vi "Acquire Data using 5772 (DRAM_sim).vi"() -> ()   [LabVIEW 2012]
uses:
  <vilib>/Platform/TimedLoop/XDataNode/XDataNode.xnode
  <vilib>/Platform/TimedLoop/XDataNode/nitl_modes.ctl
  <vilib>/Platform/TimedLoop/XDataNode/XDNodeRunTimeDep.lvlib
  <vilib>/Platform/TimedLoop/XDataNode/wakeup.ctl
  <vilib>/Platform/TimedLoop/XDataNode/timing_clust.ctl
  <vilib>/rvi/FXPMathLib/basic elements/FxpDiscreteDelay/XNode/nifxpmath_DiscreteDelay.xnode
  <userlib>/FPGA Library/Code Development/DRAM/RF-RIO/FIFO/FIFO/FPGA/FIFO.lvlib
  <userlib>/Fast OCT/Debug/Version 1/Channel Data/Data from Channel 0 and Channel 1.vi
  <userlib>/Fast OCT/Debug/Version 1/Globals/Controls.vi
panel:
  out "Data 2":i16(graph)
  out "Data":i16(graph)
  out "Record Count":u32
  out "U256s from DRAM FIFO":u32
  out "U256s to DRAM FIFO":u32
  out "Host FIFO Timed Out?":bool
  out "U64s to Host":u32
  out "U256s Acquired":u32
  in  "DRAM Arbiter Config":T1={"write grant time (clocks)"=256, "read grant time (clocks)"=256}
  in  "DRAM FIFO Depth":u8(ring)=20 items=["4"=2, "8"=3, "16"=4, "32"=5, "64"=6, "128"=7, "256"=8, "512"=9, "1024"=10, "2048"=11, "4096"=12, "8192"=13, "16384"=14, "32768"=15, "65536"=16, "131072"=17, "262144"=18, "524288"=19, "1048576"=20, "2097152"=21, "4194304"=22, "8388608"=23, "16777216"=24, "33554432"=25, "67108864"=26, "134217728"=27, "268435456"=28, "536870912"=29, "1073741824"=30, "2147483648"=31, "4294967296"=32]
  in  "Record Parameters":T2={"Load Record Parameters?"=FALSE, "Pre Trigger Samples"=2, "Post Trigger Samples"=1000, "Trigger Hold Off"=0, "Record Count"=1} {"Pre Trigger Samples" min=2}
  out "IO Module Status":T3
  out "Host FIFO Timed Out?":bool
  in  "Software Trigger":bool
  in  "Trigger Type":T4(ring)=enum."Software Trigger"
  in  "Arm Acquisition Engine":bool
  # "Digitial Trigger Input:\nPXI_Trig0 or DIO 0 on CB Front Panel"
  # "Interactive Mode Instructions\n1) Run the Emulation Mode VI for Stimulus\n1) Click on acq.Initiate, First to False and Then to True\n2) Click on Host Trigger"
  # "Status"
  # "Acquisition Engine"
  # "Acquisition Status"
  # "Record Parameters"
  # "Memory Configuration"
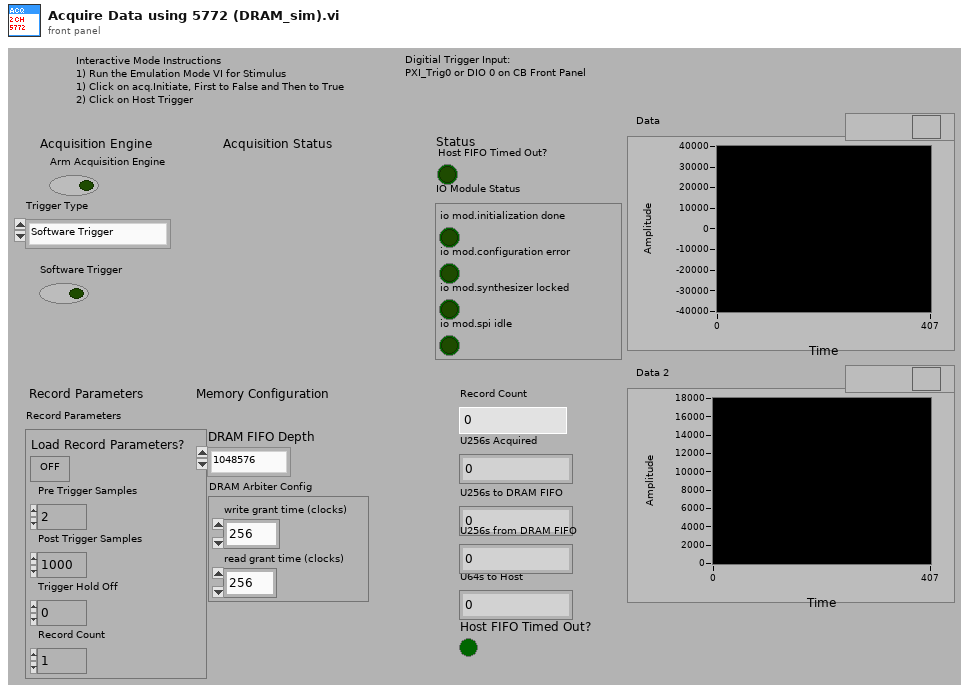
[diagram p1: front panel]
types:
  T1 = cluster{"write grant time (clocks)":u16, "read grant time (clocks)":u16}
  T2 = cluster{"Load Record Parameters?":bool, "Pre Trigger Samples":u32, "Post Trigger Samples":u32, "Trigger Hold Off":u32, "Record Count":u32}
  T3 = cluster{"io mod.initialization done":bool, "io mod.configuration error":bool, "io mod.synthesizer locked":bool, "io mod.spi idle":bool}
  T4 = enum8{"Immediate Trigger", "Software Trigger", "External Digital Trigger", "Analog Trigger"}
  T5 = typedef "XDNodeRunTimeDep.lvlib/timing_clust.ctl" = cluster{"Expected End [f-1]":u64, "Actual End [f-1]":u64, "Finished Late? [f-1]":bool, "Expected End [i-1]":u64, "Actual End [i-1]":u64, "Finished Late? [i-1]":bool, "Expected Start [i]":u64, "Actual Start [i]":u64, "Expected Start [f]":u64, "Actual Start [f]":u64, "Source Name":string, "Structure Name":string, "Period":i64, "Deadline":i64, "Offset":i64, "Start":i64, "Priority":i32, "Timeout":i32, "Mode":T6, "Wakeup Reason":T7, "Error":errorcluster, "Source Type":string, "Secondary Source Type":string, "Global End Time":u64, "Global Start Time":u64, "Frame Duration":u64, "Iteration Duration":u64, "Assigned CPU":i32, "I/O Scan Engine Mode":u32}
  T6 = typedef "XDNodeRunTimeDep.lvlib/nitl_modes.ctl" = enum32{"No Change", "Process missed periods, maintain original phase", "Discard missed periods, maintain original phase", "Process missed periods, ignore original phase", "Discard missed periods, ignore original phase"}
  T7 = typedef "XDNodeRunTimeDep.lvlib/wakeup.ctl" = enum32{"Normal", "Aborted", "Asynchronous wakeup", "Timing source error", "Timed loop error", "Timeout"}
  T8 = cluster{"fifo1 memory":refnum<k21>, "fifo2 memory":refnum<k21>}
  T9 = cluster{"Data 0":u64, "Data 1":u64, "Data 2":u64, "Data 3":u64}
  T10 = cluster{"Output":cluster{"Data 0":u64, "Data 1":u64, "Data 2":u64, "Data 3":u64}, "Output Valid":bool}
  T11 = typedef "Data Type (256).ctl" = cluster{"Bank0. High":u64, "Bank0. Low":u64, "Bank1. High":u64, "Bank1. Low":u64}
  T12 = typedef "acqEngineStates v1.ctl" = cluster{"Triggered":bool, "TrigArmed":bool, "RdyForArm":bool, "Reserved":bool}
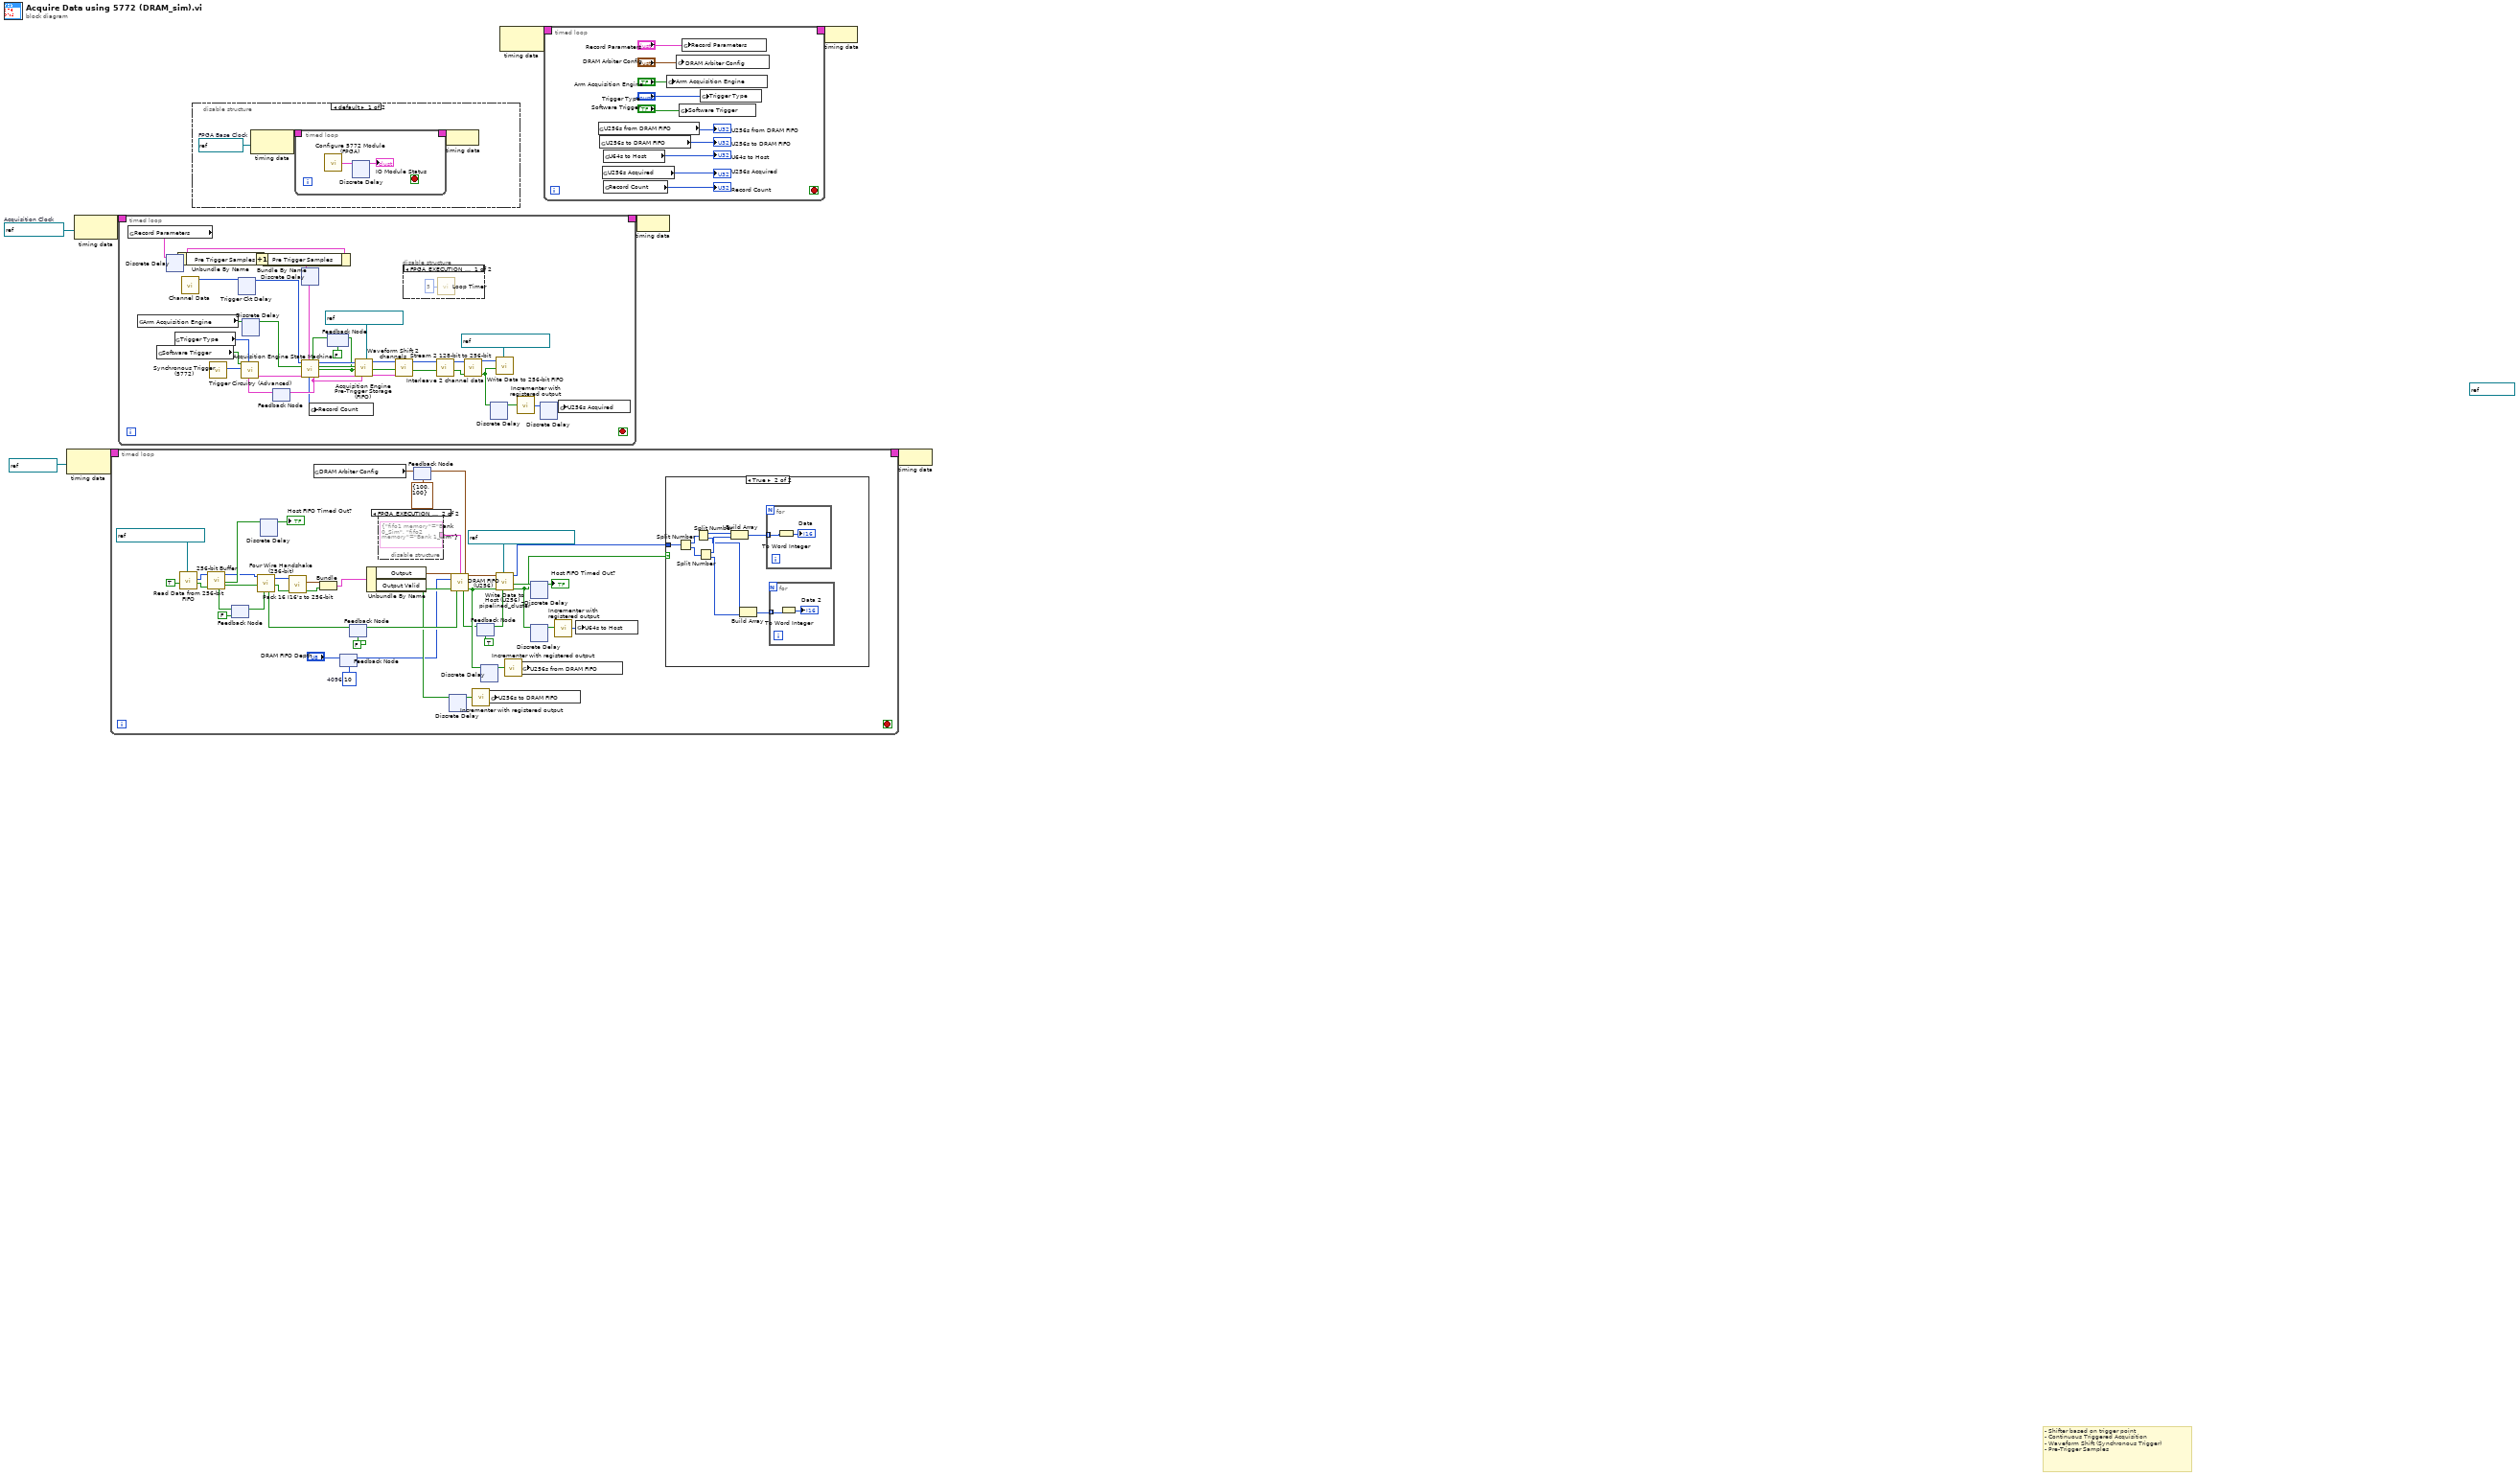
[diagram p0: block diagram]
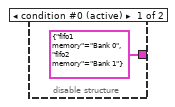
[diagram p4: hidden frame]
diagram:
  (unwired) refnum<k21> "To Host" ("FIFO In")
  w6 = refnum<k21> "ADC Clock Div 4"  # Acquisition Clock
  # "- Shifter based on trigger point\n- Continuous Triggered Acquisition\n- Waveform Shift (Synchronous Trigger)\n- Pre-Trigger Samples"
  n1 = node-c288(refnum<k21> "110MHz" ("Source Name")) -> (w5:T5)
  n2 = node-c288(w6) -> (w8:T5)
  n3 = timed-loop {
    timing: w5 -> [_]
    timing-out: [_] -> w4
    stop <- _ stop-if-true
    w28 = u8 10  # 4096
    n4 = call <userlib>:"Read Data from 256-bit FIFO.vi"("FIFO In"=refnum<k21> "FromAcqLoopU256", "Get New Data?"=TRUE) -> ("Data Valid"=w27:bool, "FIFO Data"=w26:i16[])  [unwired: 8 in]
    n5 = feedback #1(FALSE ("ready for input")) -> (w16:bool)
    n6 = call <userlib>:"256-bit Buffer.vi"("Ready for Output"=w16, "Input Valid"=w27, "Input"=w26) -> ("Output Valid"=w20:bool, "Ever Timed Out?"=w24:bool, "Output"=w19:i16[])  [unwired: 6 in]
    n7 = xnode "Discrete Delay"("D"=w24) -> ("Q"=→"Host FIFO Timed Out?":bool)
    n8 = global read "Controls.vi" "DRAM Arbiter Config"() -> (w14:T1)
    n9 = feedback-in #2("DRAM FIFO Depth") -> ()
    n10 = feedback #2(w28) -> (w29:u8)
    n11 = feedback #3(FALSE ("Ready for Input")) -> (w18:bool)
    n12 = call <userlib>:"Four Wire Handshake (256-bit).vi"("ready for output"=w18, "data valid"=w20, "Data In"=w19) -> ("valid out"=w21:bool, "Data Out"=w22:i16[], "ready for input"=w17:bool)  [unwired: 5 in, 1 out]
    n13 = feedback-in #1(w17) -> ()
    n14 = call <userlib>:"Pack 16 I16's to 256-bit.vi"("Data Valid"=w21, "Input"=w22) -> ("Output Valid"=w39:bool, "Output"=w40:T9)  [unwired: 7 in, 1 out]
    n15 = Bundle("Output"=w40, "Output Valid"=w39) -> (w36:T10)  [unwired: 1 in]
    n16 = Unbundle By Name(w36) -> ("Output"=w38:T9, "Output Valid"=w37:bool)
    n17 = disable-structure shown="FPGA_EXECUTION_MODE==DEV_COMPUTER_SIM_IO" {
      disable-tunnel: [T8 {"fifo1 memory"="Bank 0", "fifo2 memory"="Bank 1"} ("Memory") T8 {"fifo1 memory"="Bank 0_Sim", "fifo2 memory"="Bank 1_Sim"} ("Memory")] -> w50
      frame condition #0 (active) {
      }
      frame condition #1 {
      }
    }
    n18 = feedback-in #4(w14) -> ()
    n19 = feedback #4(T1 {"write grant time (clocks)"=100, "read grant time (clocks)"=100} ("DRAM Arbiter Config")) -> (w30:T1)
    n20 = xnode "Discrete Delay"("D"=w37) -> ("Q"=w33:bool)
    n21 = call <userlib>:"Incrementer with registered output.vi"("INC?"=w33) -> ("count"=w11:u32)  [unwired: 4 in]
    n22 = feedback #5(TRUE ("Ready For Input")) -> (w42:bool)
    n23 = call <userlib>:"DRAM FIFO (U256).vi"("Input Data"=w38, "Memory"=w50, "arbiter configuration"=w30, "fifo depth"=w29, "input valid"=w37, "ready for output"=w42) -> ("Output Data"=w47:T11, "Ready for Input"=w49:bool, "Output Valid"=w44:bool)  [unwired: 4 in, 3 out]
    n24 = feedback-in #3(w49) -> ()
    n25 = xnode "Discrete Delay"("D"=w44) -> ("Q"=w34:bool)
    n26 = global write "Controls.vi" "U256s to DRAM FIFO"(w11) -> ()
    n27 = call <userlib>:"Write Data to Host (U256) _pipelined_cluster.vi"("FIFO In"=refnum<k21> "FPGA to Host FIFO (U64)" ("FIFO Out"), "Input Valid"=w44, "Input"=w47) -> ("Valid Data to Host"=w10:bool, "Timed Out?"=w46:bool, "Data to Host"=w9:u64, "Ready For Input"=w43:bool)  [unwired: 5 in]
    n28 = feedback-in #5(w43) -> ()
    n29 = call <userlib>:"Incrementer with registered output.vi"("INC?"=w34) -> ("count"=w12:u32)  [unwired: 4 in]
    n30 = global write "Controls.vi" "U256s from DRAM FIFO"(w12) -> ()
    n31 = xnode "Discrete Delay"("D"=w46) -> ("Q"=→"Host FIFO Timed Out?":bool)
    n32 = xnode "Discrete Delay"("D"=w10) -> ("Q"=w35:bool)
    n33 = call <userlib>:"Incrementer with registered output.vi"("INC?"=w35) -> ("count"=w13:u32)  [unwired: 4 in]
    n34 = global write "Controls.vi" "U64s to Host"(w13) -> ()
    n35 = case shown="True" w10 {
      tunnel: w9 -> [_ w61]
      frame False {
      }
      frame True {
        n36 = Split Number(x=w61) -> (hi(x)=w60:u32, lo(x)=w59:u32)
        n37 = Split Number(x=w60) -> (hi(x)=w58:u16, lo(x)=w55:u16)
        n38 = Split Number(x=w59) -> (hi(x)=w57:u16, lo(x)=w54:u16)
        n39 = Build Array(w58, w57) -> (w56:u16[])
        n40 = Build Array(w55, w54) -> (w53:u16[])
        n41 = for {
          tunnel: w56 -> [w65] mode=indexing
          n42 = To Word Integer(number=w65) -> (16bit integer=→"Data":i16)
        }
        n43 = for {
          tunnel: w53 -> [w62] mode=indexing
          n44 = To Word Integer(number=w62) -> (16bit integer=→"Data 2":i16)
        }
      }
    }
  }
  n45 = timed-loop {
    timing: w8 -> [_]
    timing-out: [_] -> w7
    stop <- _ stop-if-true
    n46 = global read "Controls.vi" "Record Parameters"() -> (w76:T2)
    n47 = global read "Controls.vi" "Arm Acquisition Engine"() -> (w71:bool)
    n48 = global read "Controls.vi" "Software Trigger"() -> (w72:bool)
    n49 = xnode "Discrete Delay"("D"=w76) -> ("Q"=w80:T2)
    n50 = global read "Controls.vi" "Trigger Type"() -> (w73:T4)
    n51 = Unbundle By Name(w80) -> ("Pre Trigger Samples"=w93:u32)
    n52 = call-poly <userlib>:"Channel Data.vi"() -> ("Channels Data"=w106:i16[])  [unwired: 11 in]
    n53 = call <userlib>:"Synchronous Trigger (5772).vi"() -> ("Trigger"=w99:u8)  [unwired: 9 in, 2 out]
    n54 = xnode "Trigger Ckt Delay"("D"=w106) -> ("Q"=w90:i16[])
    n55 = xnode "Discrete Delay"("D"=w71) -> ("Q"=w77:bool)
    n56 = Increment(x=w93) -> (x+1=w92:u32)
    n57 = Bundle By Name(cluster=w80, "Pre Trigger Samples"=w92) -> (w91:T2)
    n58 = feedback #6() -> (w103:T12)  [unwired: 1 in]
    n59 = call <userlib>:"Trigger Circuitry (Advanced).vi"("State Machine State"=w103, "Trigger Type"=w73, "Digital Trigger Value"=w99, "Software Trigger from Host"=w72) -> ("Trigger Info"=w97:cluster{"Trigger":bool, "Trig Offset":u8})  [unwired: 5 in, 2 out]
    n60 = xnode "Discrete Delay"("D"=w91) -> ("Q"=w79:T2)
    n61 = feedback #7(FALSE ("flushed")) -> (w102:bool)
    n62 = call <userlib>:"Acquisition Engine State Machine.vi"("Start Next Record"=w102, "Record Parameters"=w79, "Trigger Info"=w97, "Arm Acquisition Engine"=w77, "Input"=w90) -> ("Trigger Info"=w104:cluster{"Trigger":bool, "Trig Offset":u8}, "PostTrigComplete"=w70:bool, "AcqInProgress"=w96:bool, "Output"=w105:i16[], "States"=w95:T12, "Record Count"=w75:u32)  [unwired: 1 in]
    n63 = feedback-in #6(w95) -> ()
    n64 = global write "Controls.vi" "Record Count"(w75) -> ()
    n65 = feedback-in #7(w70) -> ()
    n66 = call <userlib>:"Acquisition Engine Pre-Trigger Storage (FIFO).vi"("FIFO Out"=refnum<k21> "HistoryFIFOU128", "states"=w95, "Trigger Info"=w104, "PostTrigComplete"=w70, "AcqInProgress"=w96, "Input Data"=w105) -> ("Trigger Info"=w100:cluster{"Trigger":bool, "Trig Offset":u8}, "Output Valid"=w88:bool, "Output Data"=w89:i16[])  [unwired: 2 in, 1 out]
    n67 = call <userlib>:"Waveform Shift 2 channels.vi"("Trigger Info"=w100, "Input Valid"=w88, "Input Data"=w89) -> ("Output Valid"=w87:bool, "Shifted Output Data"=w85:i16[])  [unwired: 5 in, 2 out]
    n68 = disable-structure shown="FPGA_EXECUTION_MODE==DEV_COMPUTER_SIM_IO" {
      frame condition #0 {
        n69 = call "Loop Timer"("Count(mSec)"=u32 5) -> ()  [unwired: 1 out]
      }
      frame condition #1 (active) {
      }
    }
    n70 = call <userlib>:"Interleave 2 channel data.vi"("Input Valid"=w87, "Raw Data"=w85) -> ("Output Valid"=w83:bool, "Interleaved Data"=w84:i16[])  [unwired: 8 in]
    n71 = call <userlib>:"Stream 2 128-bit to 256-bit.vi"("Input Valid"=w83, "Input Data"=w84) -> ("Output Valid"=w81:bool, "Output Data"=w82:i16[])  [unwired: 8 in]
    n72 = xnode "Discrete Delay"("D"=w81) -> ("Q"=w78:bool)
    n73 = call <userlib>:"Write Data to 256-bit FIFO.vi"("FIFO In"=refnum<k21> "FromAcqLoopU256", "Input Valid"=w81, "Data"=w82) -> ()  [unwired: 7 in, 2 out]
    n74 = call <userlib>:"Incrementer with registered output.vi"("INC?"=w78) -> ("count"=w94:u32)  [unwired: 4 in]
    n75 = xnode "Discrete Delay"("D"=w94) -> ("Q"=w74:u32)
    n76 = global write "Controls.vi" "U256s Acquired"(w74) -> ()
  }
  n77 = disable-structure shown="default" {
    frame condition #0 (active) {
      w110 = refnum<k21> "40 MHz"  # FPGA Base Clock
      n78 = node-c288(w110) -> (w112:T5)
      n79 = timed-loop {
        timing: w112 -> [_]
        timing-out: [_] -> w111
        stop <- _ stop-if-true
        n80 = call <userlib>:"Configure 5772 Module (FPGA).vi"() -> ("IO Module Status"=w114:T3)  [unwired: 5 in]
        n81 = xnode "Discrete Delay"("D"=w114) -> ("Q"=→"IO Module Status":T3)
      }
      n82 = node-c288(w111) -> ()
    }
    frame condition #1 {
    }
  }
  n83 = node-c288() -> (w2:T5)  [unwired: 1 in]
  n84 = timed-loop {
    timing: w2 -> [_]
    timing-out: [_] -> w1
    stop <- _ stop-if-true
    n85 = global read "Controls.vi" "U256s from DRAM FIFO"() -> (→"U256s from DRAM FIFO":u32)
    n86 = global read "Controls.vi" "U256s to DRAM FIFO"() -> (→"U256s to DRAM FIFO":u32)
    n87 = global read "Controls.vi" "U256s Acquired"() -> (→"U256s Acquired":u32)
    n88 = global read "Controls.vi" "U64s to Host"() -> (→"U64s to Host":u32)
    n89 = global read "Controls.vi" "Record Count"() -> (→"Record Count":u32)
    n90 = global write "Controls.vi" "Arm Acquisition Engine"("Arm Acquisition Engine") -> ()
    n91 = global write "Controls.vi" "DRAM Arbiter Config"("DRAM Arbiter Config") -> ()
    n92 = global write "Controls.vi" "Software Trigger"("Software Trigger") -> ()
    n93 = global write "Controls.vi" "Record Parameters"("Record Parameters") -> ()
    n94 = global write "Controls.vi" "Trigger Type"("Trigger Type") -> ()
  }
  n95 = node-c288(w7) -> ()
  n96 = node-c288(w1) -> ()
  n97 = node-c288(w4) -> ()
